vi "Wait for cmd execution state.vi"(0 "quitscan":T2, 1 "stop waiting for response":T2, 5 "TCP Ports":refnum<k5>[](array[refnum]), 7 "> Cmd Sent >":string, 9 "Expected slow response":string, 11 "last udp comm ok":bool, 12 "ms time command start":u32) -> (2 "update active variable":bool, 3 "slow response out":string, 4 "Boolean":bool, 6 "Next steps":T1, 8 "variable value":string, 10 "Numeric 2":u32, 14 "Visible":bool, 15 "Numeric":u32)   [LabVIEW 2018]
uses:
  general button2.ctl
  wait for cmd exec next steps.ctl
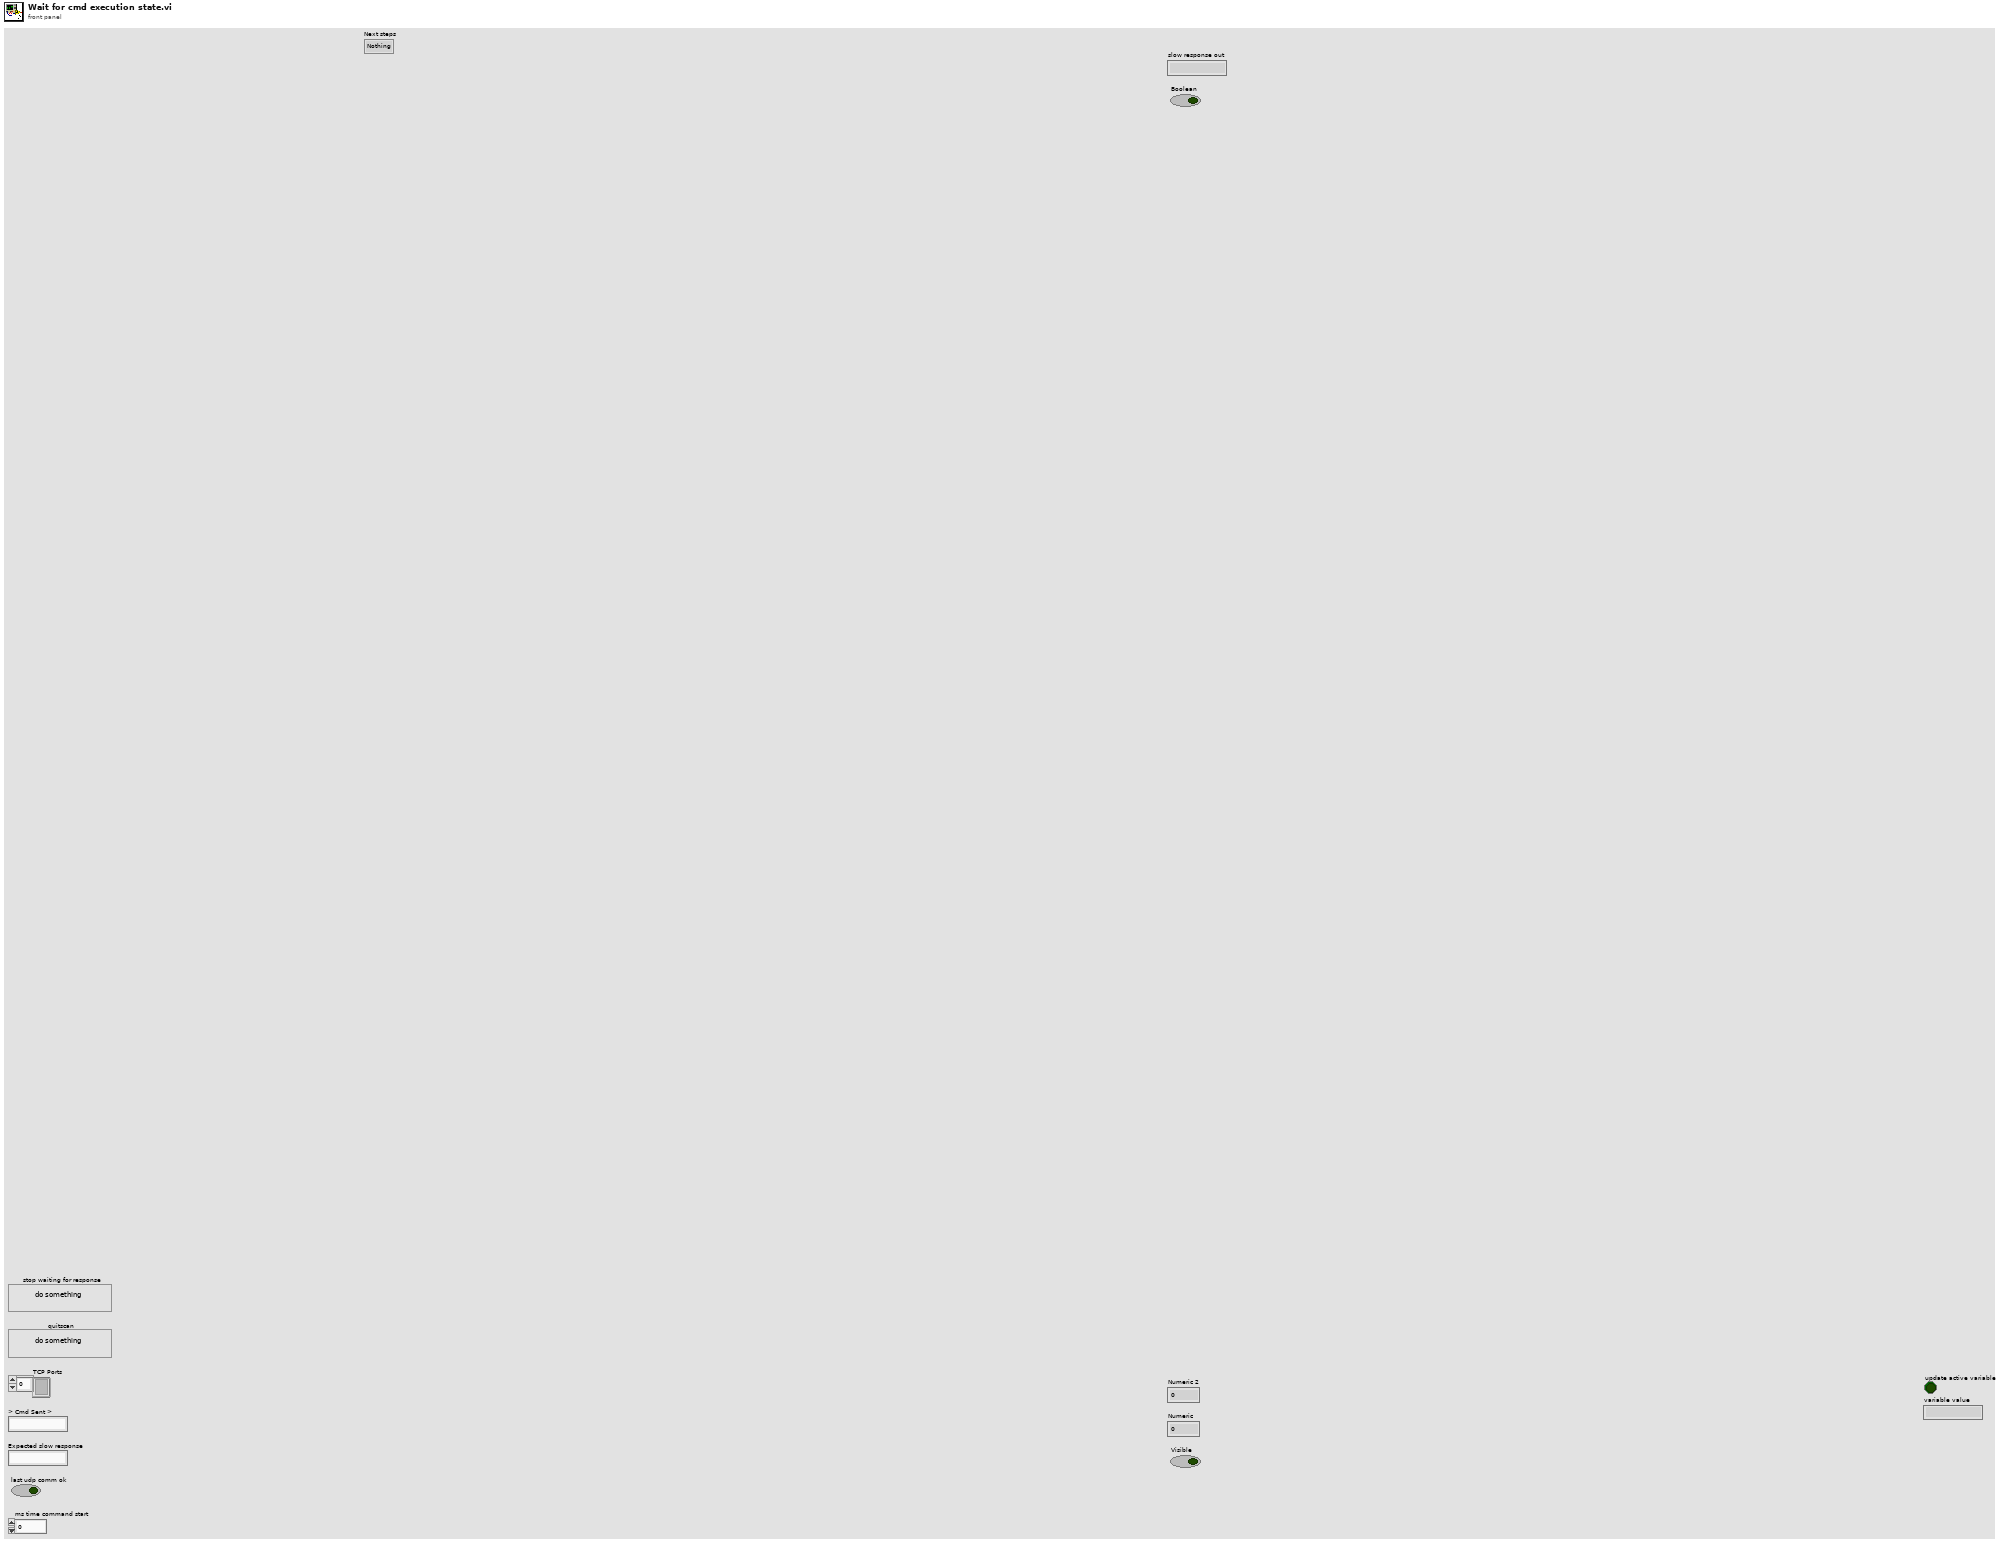
[diagram p1: front panel]
types:
  T1 = typedef "wait for cmd exec next steps.ctl" = enum16{"Nothing", "UDP only", "TCP", "TCP and check again", "check again"}
  T2 = typedef "general button2.ctl" = bool
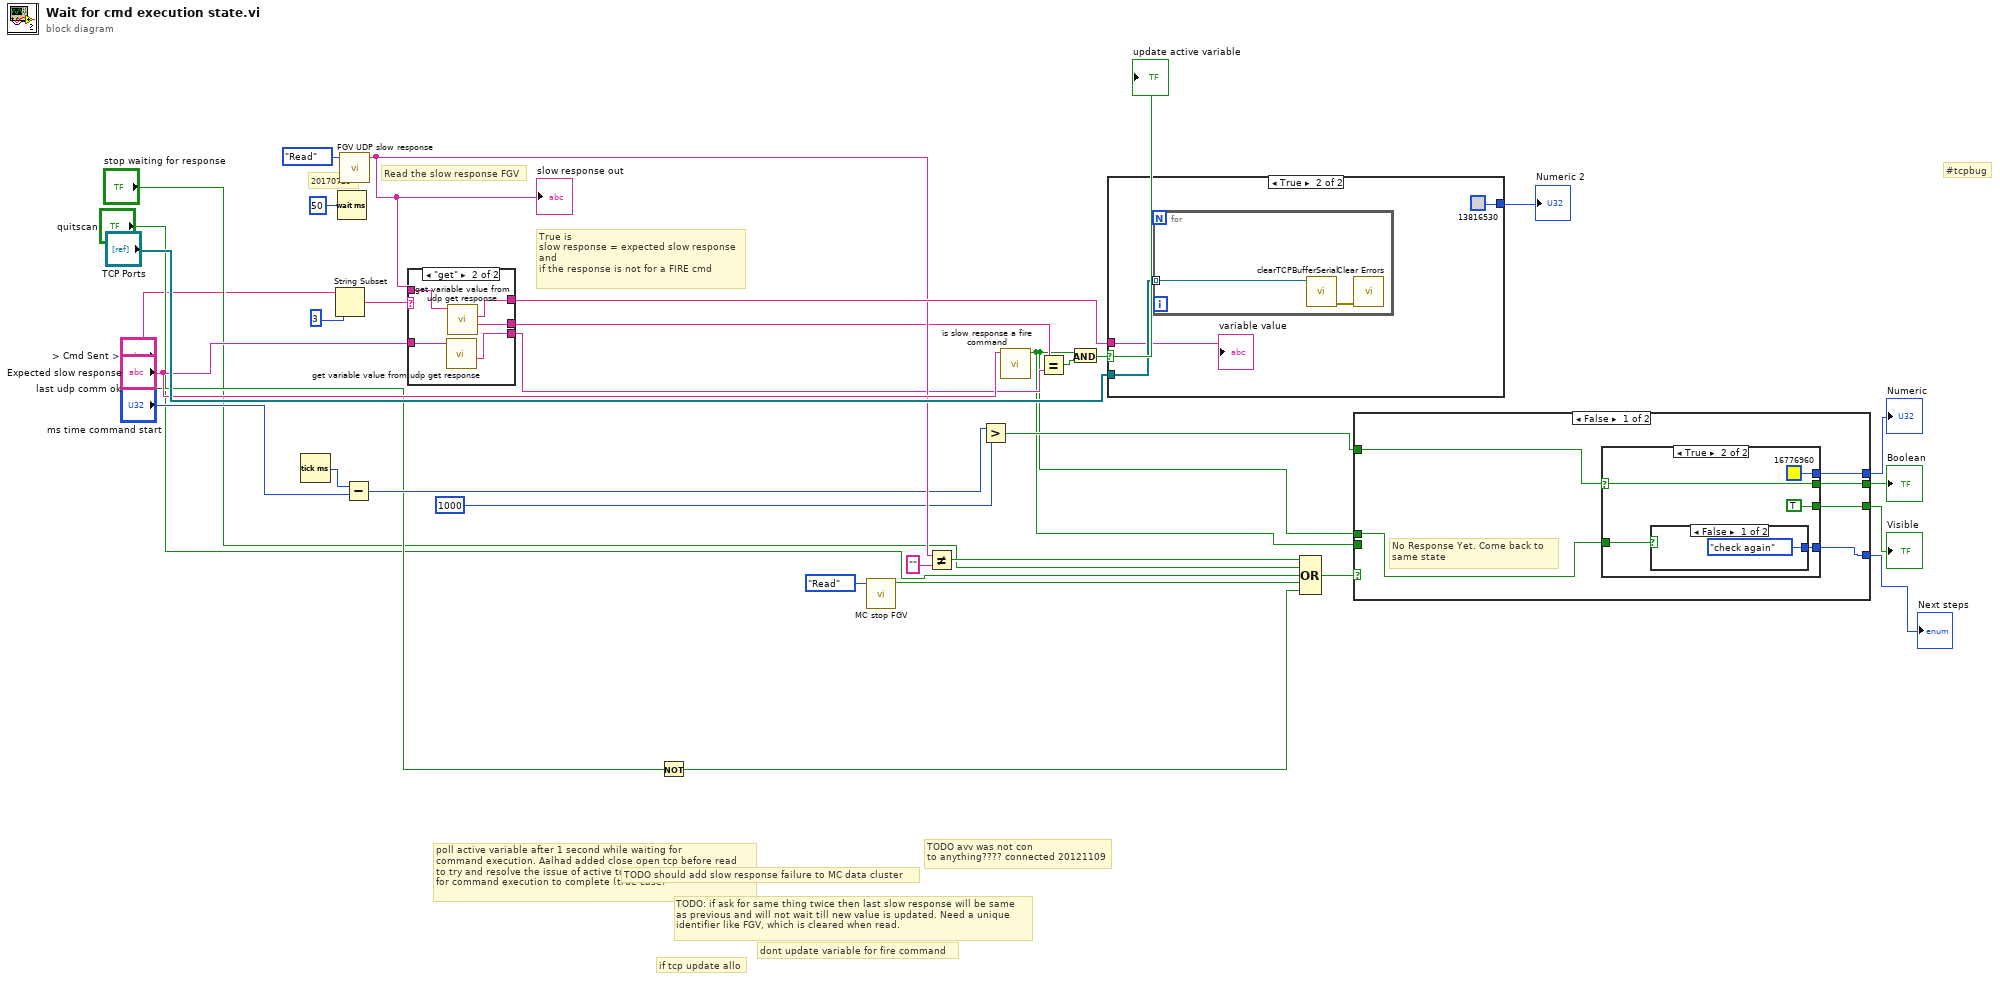
[diagram p0: block diagram]
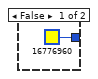
[diagram p2: hidden frame]
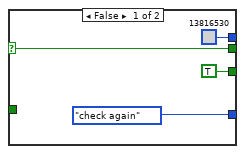
[diagram p3: hidden frame]
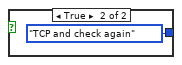
[diagram p4: hidden frame]
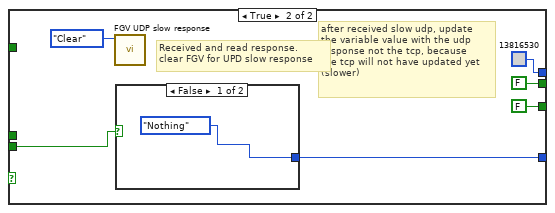
[diagram p5: hidden frame]
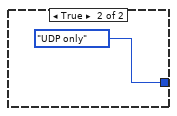
[diagram p6: hidden frame]
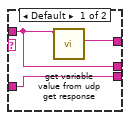
[diagram p7: hidden frame]
diagram:
  # "#tcpbug"
  # "20170729"
  # "if tcp update allo"
  # "dont update variable for fire command"
  # "poll active variable after 1 second while waiting for \ncommand execution. Aalhad added close open tcp before read\nto try and resolve the issue of active tcp update while waiting \nfor command execution to complete (true case)"
  # "True is \nslow response = expected slow response\nand\nif the response is not for a FIRE cmd"
  # "Read the slow response FGV"
  # "TODO avv was not con\nto anything???? connected 20121109"
  # "TODO: if ask for same thing twice then last slow response will be same\nas previous and will not wait till new value is updated. Need a unique\nidentifier like FGV, which is cleared when read."
  # "TODO should add slow response failure to MC data cluster"
  n1 = Tick Count (ms)() -> (millisecond timer value=w17:u32)
  n2 = String Subset(string="> Cmd Sent >", length (rest)=3 ("offset (0)")) -> (substring=w14:string)  [unwired: 1 in]
  n3 = Wait (ms)(milliseconds to wait=u32 50) -> ()  [unwired: 1 out]
  n4 = call "FGV UDP slow response.vi"("Function"=enum16{"Read", "Write", "Clear"}."Read") -> ("slow response out"=w23:string)  [unwired: 9 in, 1 out]
  "slow response out" <- w23
  n5 = Subtract(x=w17, y="ms time command start") -> (x-y=w19:u32)
  n6 = case shown="\"get\"" w14 {
    tunnel: "Expected slow response" -> [w36 w41]
    tunnel: [w36 w40] -> w3
    tunnel: [w35 w39] -> w22
    tunnel: w23 -> [w35 w38]
    tunnel: [w34 w37] -> w27
    frame Default {
      n7 = call "get variable value from udp get response.vi"("slow get response or tcp response"=w35) -> ("variable value"=w34:string)  [unwired: 4 in, 2 out]
    }
    frame "get" {
      n8 = call "get variable value from udp get response.vi"("slow get response or tcp response"=w41) -> ("slow get response without value"=w40:string)  [unwired: 4 in, 2 out]
      n9 = call "get variable value from udp get response.vi"("slow get response or tcp response"=w38) -> ("slow get response without value"=w39:string, "variable value"=w37:string)  [unwired: 4 in, 1 out]
    }
  }
  n10 = Not(x="last udp comm ok") -> (.not. x?=w16:bool)
  n11 = call "MC stop FGV.vi"("Function"=enum16{"Read", "Write", "Clear"}."Read") -> ("Stop out"=w11:bool)  [unwired: 9 in, 1 out]
  n12 = Not Equal?(x=w23, y="" ("Last Slow response")) -> (x != y?=w25:bool)
  n13 = Greater?(x=w19, y=u32 1000) -> (0:w21:bool)
  n14 = call "is slow response a fire command.vi"("Expected slow response"="Expected slow response") -> ("False is Fire cmd"=w1:bool)  [unwired: 10 in]
  n15 = Equal?(x=w22, y=w3) -> (x = y?=w28:bool)
  n16 = And(x=w1, y=w28) -> (x .and. y?=w29:bool)
  "update active variable" <- w29
  n17 = case shown="True" w29 {
    tunnel: w27 -> [_ w43]
    tunnel: [u32 16776960 u32 13816530] -> w26
    tunnel: "TCP Ports" -> [_ w44]
    frame False {
    }
    frame True {
      n18 = for {
        tunnel: w44 -> [w47] mode=indexing
        n19 = call "clearTCPBufferSerial.vi"("connection ID in"=w47) -> ("error out"=w46:errorcluster)  [unwired: 9 in, 1 out]
        n20 = call <vilib>:"Clear Errors.vi"("error in (no error)"=w46) -> ()  [unwired: 5 in, 2 out]
      }
      "variable value" <- w43
    }
  }
  "Numeric 2" <- w26
  n21 = Compound Arithmetic op=OR(w25, "stop waiting for response", "quitscan", w11, w16) -> (w13:T2)
  n22 = case shown="False" w13 {
    tunnel: w21 -> [w53 _]
    tunnel: [w52 FALSE] -> w24
    tunnel: [w51 u32 13816530] -> w32
    tunnel: [w50 FALSE ("Visible")] -> w33
    tunnel: w1 -> [_ w66]
    tunnel: [w49 w65] -> w2
    tunnel: w1 -> [w48 _]
    frame False {
      # "No Response Yet. Come back to \nsame state"
      n23 = case shown="True" w53 {
        selector: w53 -> [w57 w62]
        tunnel: [w57 w62] -> w52
        tunnel: [u32 13816530 u32 16776960] -> w51
        tunnel: [TRUE ("Visible") TRUE ("Visible")] -> w50
        tunnel: [wait_for_cmd_exec_next_steps."check again" ("Next steps") w59] -> w49
        tunnel: w48 -> [_ w58]
        frame False {
        }
        frame True {
          n24 = case shown="False" w58 {
            tunnel: [wait_for_cmd_exec_next_steps."check again" ("Next steps") wait_for_cmd_exec_next_steps."TCP and check again" ("Next steps")] -> w59
            frame False {
            }
            frame True {
            }
          }
        }
      }
    }
    frame True {
      # "after received slow udp, update\nthe variable value with the udp\nresponse not the tcp, because\nthe tcp will not have updated yet\n(slower)"
      # "Received and read response.\nclear FGV for UPD slow response"
      n25 = call "FGV UDP slow response.vi"("Function"=enum16{"Read", "Write", "Clear"}."Clear") -> ()  [unwired: 9 in, 2 out]
      n26 = case shown="False" w66 {
        tunnel: [wait_for_cmd_exec_next_steps."Nothing" ("Next steps") wait_for_cmd_exec_next_steps."UDP only" ("Next steps")] -> w65
        frame False {
        }
        frame True {
        }
      }
    }
  }
  "Visible" <- w33
  "Numeric" <- w32
  "Boolean" <- w24
  "Next steps" <- w2
